vi "Calculate Convex Point Local.vi"(0 "pdX":dbl[](array[numeric])=array[4097 elements], 1 "pnIndexPeak2":i32, 5 "pdZ":dbl[](array[numeric])=array[4097 elements], 7 "nLength":i32, 9 "pnIndexPeak1":i32, 11 "error in (no error)":errorcluster caption="错误输入（无错误）", 12 "pnIndexConvex":i32) -> (3 "pnIndexPeak2 out":i32, 4 "pdX out":dbl[](array[numeric]), 6 "pdZ out":dbl[](array[numeric]), 8 "function return":bool, 10 "pnIndexPeak1 out":i32, 14 "pnIndexConvex out":i32, 15 "error out":errorcluster caption="错误输出")   [LabVIEW 2015, in "CalculateConvexDll.lvlib"]
doc: "CALCULATE_CONVEX_DLL bool CalculateConvexPointLocal(double pdX[], double pdZ[], int nLength, int* pnIndexPeak1, int* pnIndexPeak2, int* pnIndexConvex);"
uses:
  CalculateConvexDll.lvlib
  CalculateConvexDll.dll
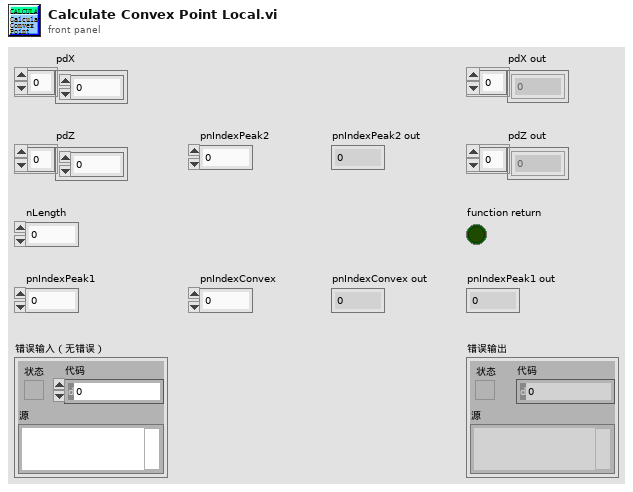
[diagram p1: front panel]
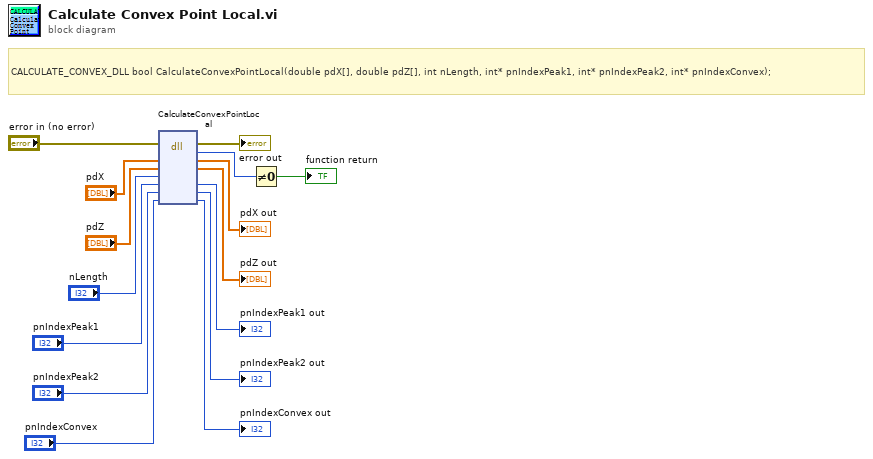
[diagram p0: block diagram]
diagram:
  # "CALCULATE_CONVEX_DLL bool CalculateConvexPointLocal(double pdX[], double pdZ[], int nLength, int* pnIndexPeak1, int* pnIndexPeak2, int* pnIndexConvex);"
  n1 = dll-call lib="D:/WNC3d/AxxonSoftware WNC 20201114/KEYENCE LJ-X8000/user/CalculateConvexDll_vis/CalculateConvexDll.*" fn="CalculateConvexPointLocal"(error in="error in (no error)", "pdX"="pdX", "pdZ"="pdZ", "nLength"="nLength", "pnIndexPeak1"="pnIndexPeak1", "pnIndexPeak2"="pnIndexPeak2", "pnIndexConvex"="pnIndexConvex") -> (error out=→"error out":errorcluster, w14:u8, "pdX"=→"pdX out":dbl[], "pdZ"=→"pdZ out":dbl[], "pnIndexPeak1"=→"pnIndexPeak1 out":i32, "pnIndexPeak2"=→"pnIndexPeak2 out":i32, "pnIndexConvex"=→"pnIndexConvex out":i32)  [unwired: 3 in, 1 out]
  n2 = Not Equal To 0?(x=w14) -> (x != 0?=→"function return":bool)
